vi "RIB Req - UDP Connect.vi"(0 "Limits File Path":path, 5 "Results File Path":path, 11 "error in":errorcluster) -> (4 "Results Data Array":string[][](array[string]), 15 "error out":errorcluster)   [LabVIEW 2024]
doc: "Template test"
uses:
  <vilib>/addons/_JKI Toolkits/State Machine/_JKI_lib_State_Machine.llb/Select State(s)_err__jki_lib_state_machine.vi
  <vilib>/DAQmx/write.llb/DAQmx Write (Digital 1D Bool 1Chan 1Samp).vi
  <vilib>/addons/_JKI Toolkits/State Machine/_JKI_lib_State_Machine.llb/Select State(s)_bool__jki_lib_state_machine.vi
  <vilib>/addons/_JKI Toolkits/State Machine/_JKI_lib_State_Machine.llb/Periodic Trigger__ogtk__JKI-SM__jki_lib_state_machine.vi
  <userlib>/_OpenG.lib/file/file.llb/Strip Path Extension - String__ogtk.vi
  <vilib>/Utility/file.llb/Read Delimited Spreadsheet (string).vi
  <vilib>/Utility/file.llb/Write Delimited Spreadsheet (string).vi
  <vilib>/DAQmx/create/channels.llb/DAQmx Create Channel (DO-Digital Output).vi
  <vilib>/DAQmx/miscellaneous.llb/DAQmx Fill In Error Info.vi
  <userlib>/_OpenG.lib/file/file.llb/openg_file.lvlib
  <userlib>/_OpenG.lib/appcontrol/appcontrol.llb/openg_application_control.lvlib
  <userlib>/_OpenG.lib/time/time.llb/openg_time.lvlib
panel:
  out "Connect":bool
  out "Connect Fail":bool
  out "Timeout (Connect Fail)":dbl(slide) scale=0.0..10.0
  out "Timeout (Connect)":dbl(slide) scale=0.0..10.0
  in  "Connect":string
  in  "Connect Fail":string
  out "Results Data 5":string[](array[string])
  out "Results Data 4":string[](array[string])
  in  "task out":refnum<k21>
  in  "UDP Read":string
  in  "connection ID":refnum<k16>
  in  "Exit":bool
  # "UDP Initialise Test"
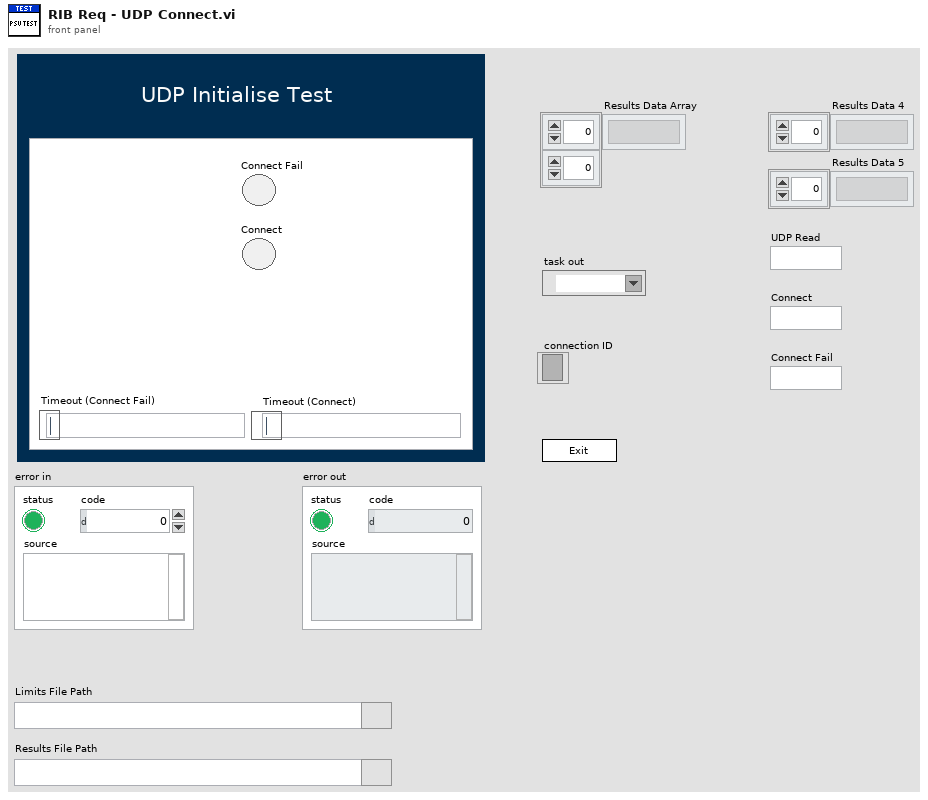
[diagram p1: front panel]
types:
  T1 = enum32{"Invalid", "Standard", "Closed", "Hidden", "Minimized", "Maximized"}
  T2 = enum32{"invalid app kind", "Development System", "Run Time System", "Student Edition", "Embedded LabVIEW", "Evaluation", "Custom"}
  T3 = typedef "FGV - Enum" = enum16{"Cleanup", "Get Data", "Open UDP", "Initialise DAQ", "Initialise I2C"}
  T4 = enum16{"Start Timer", "Get Time", "Pause", "Unpause"}
  T5 = cluster{"Core":cluster{"Current VI Reference":refnum<vi>, "Close Panel on Exit?":bool}, "Limits File Path":path, "Test Limits":string[][], "Results Data Array":string[][], "Results File Path":path, "UDP Read":string, "connection ID":refnum<k16>, "task out":refnum<k21>, "Connect Fail":string, "Connect":string}
  T6 = cluster{"Current VI Reference":refnum<vi>, "Close Panel on Exit?":bool}
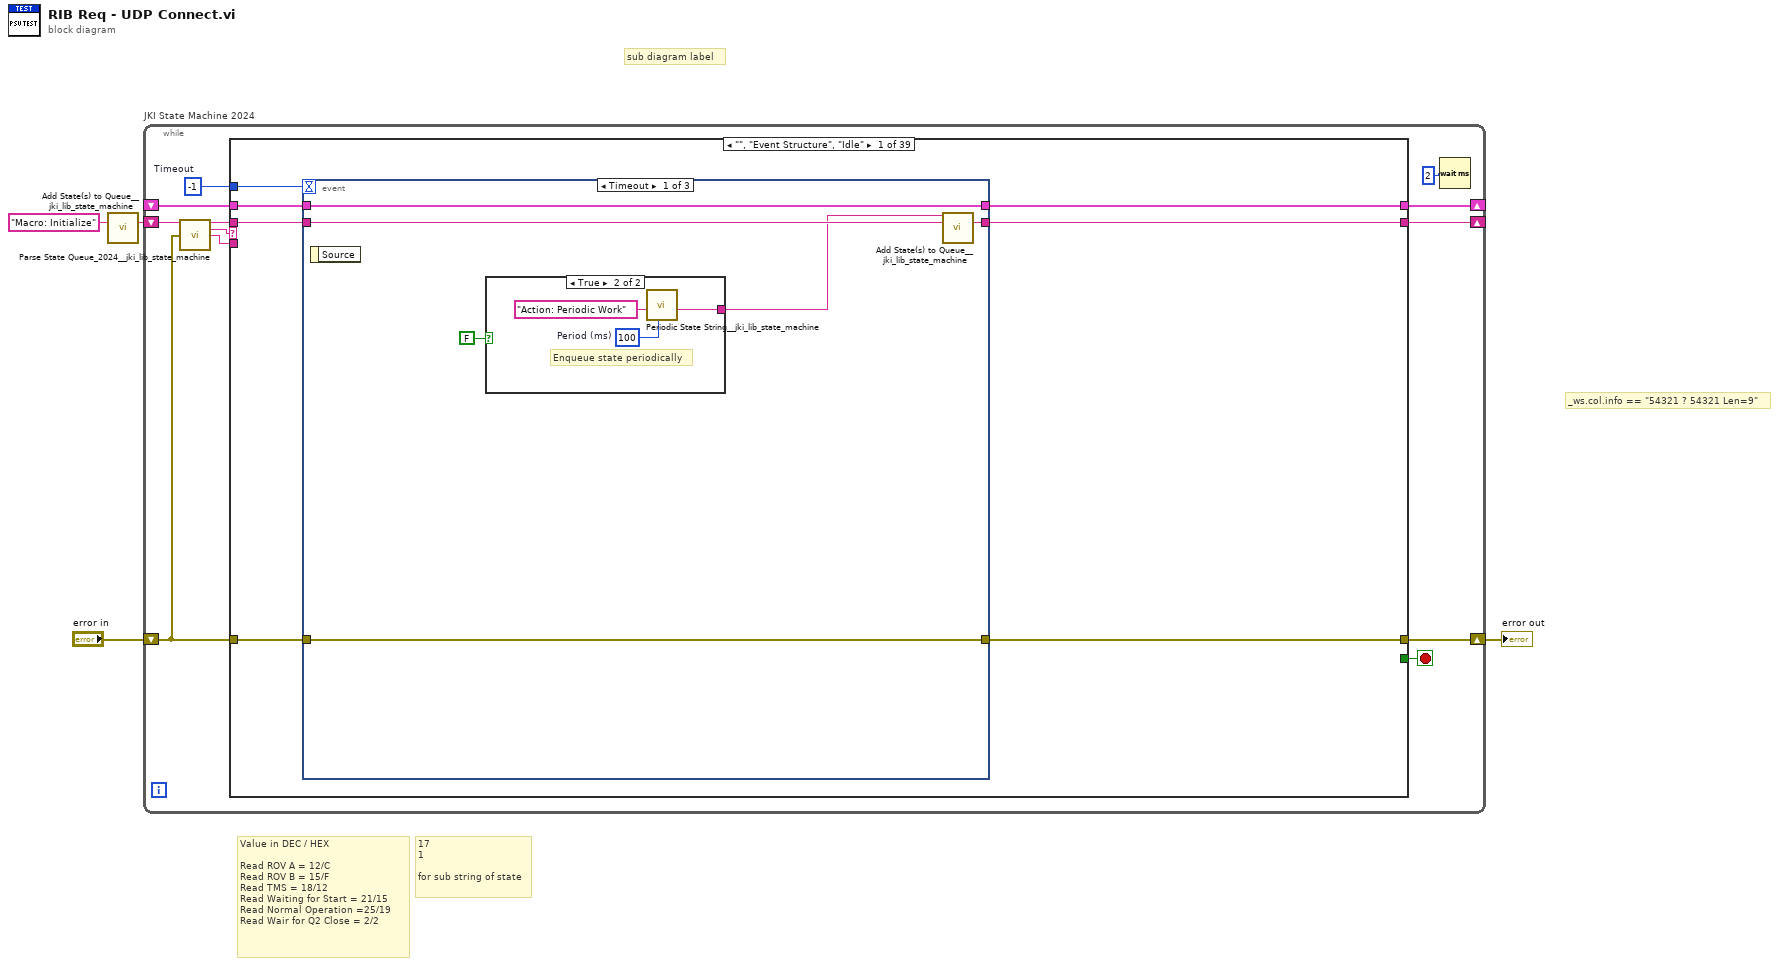
[diagram p0: block diagram]
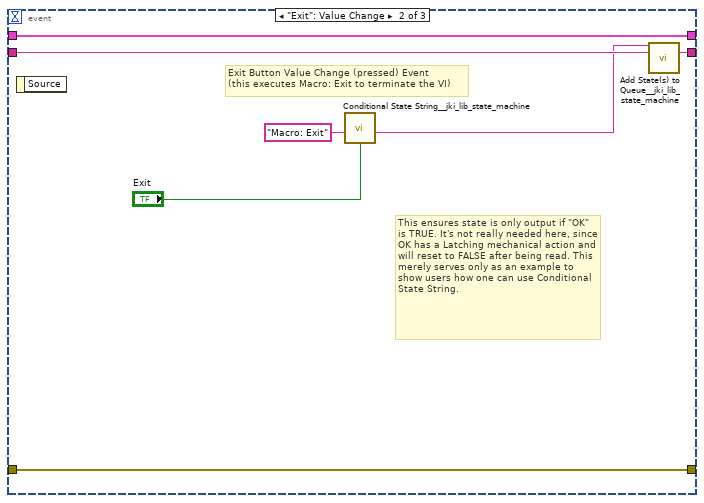
[diagram p3: hidden frame]
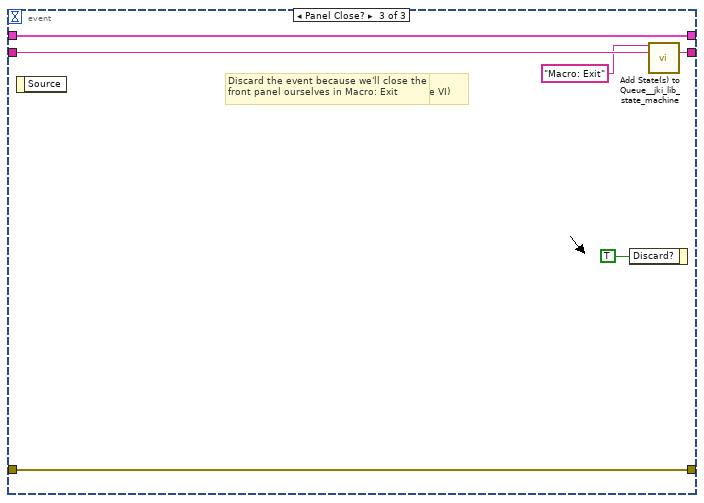
[diagram p4: hidden frame]
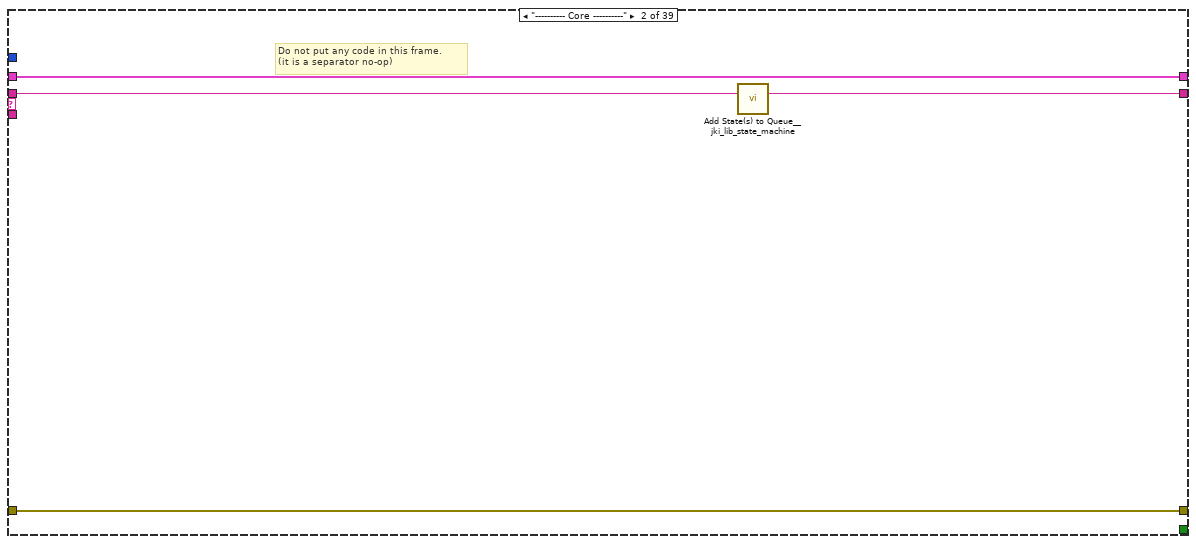
[diagram p5: hidden frame]
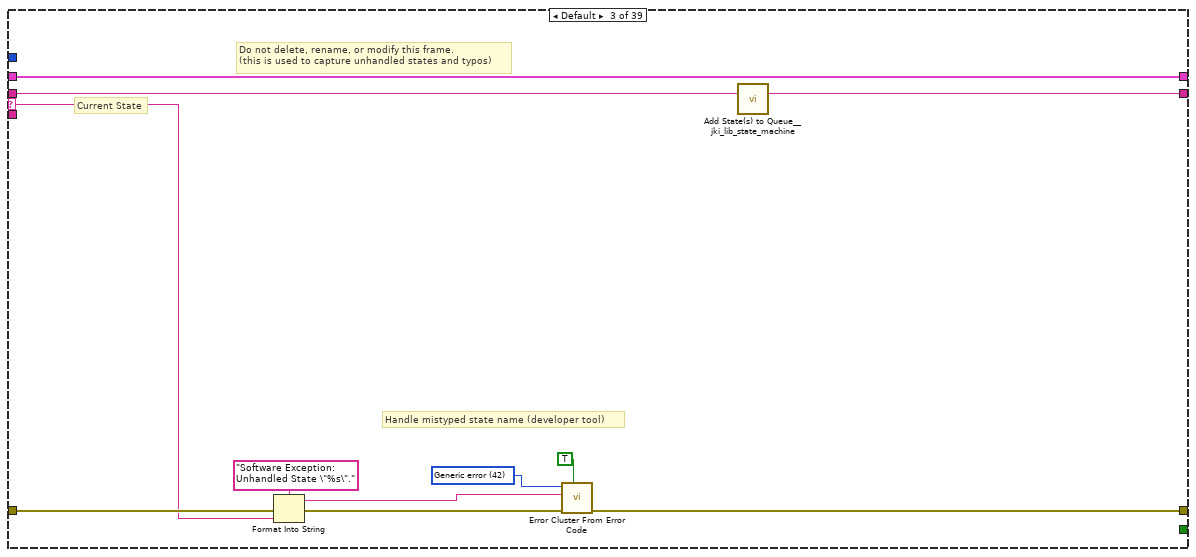
[diagram p6: hidden frame]
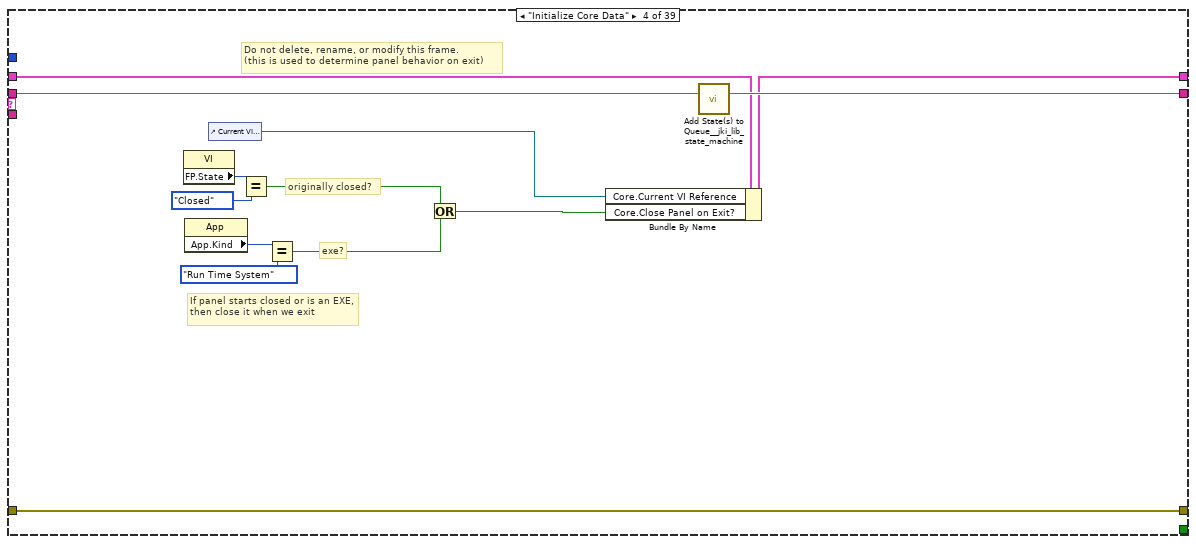
[diagram p7: hidden frame]
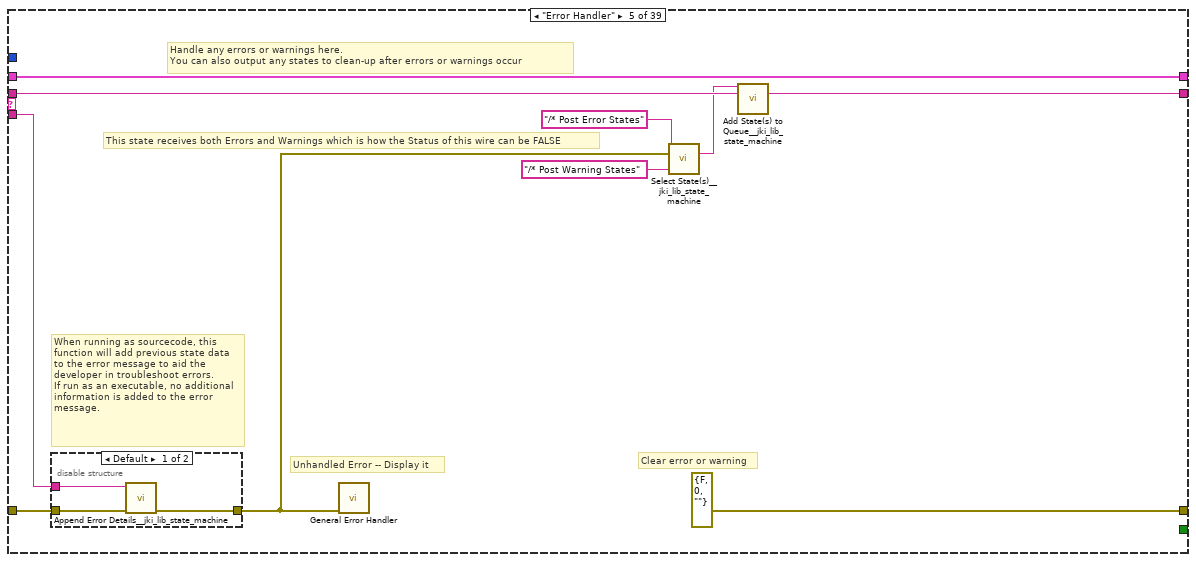
[diagram p8: hidden frame]
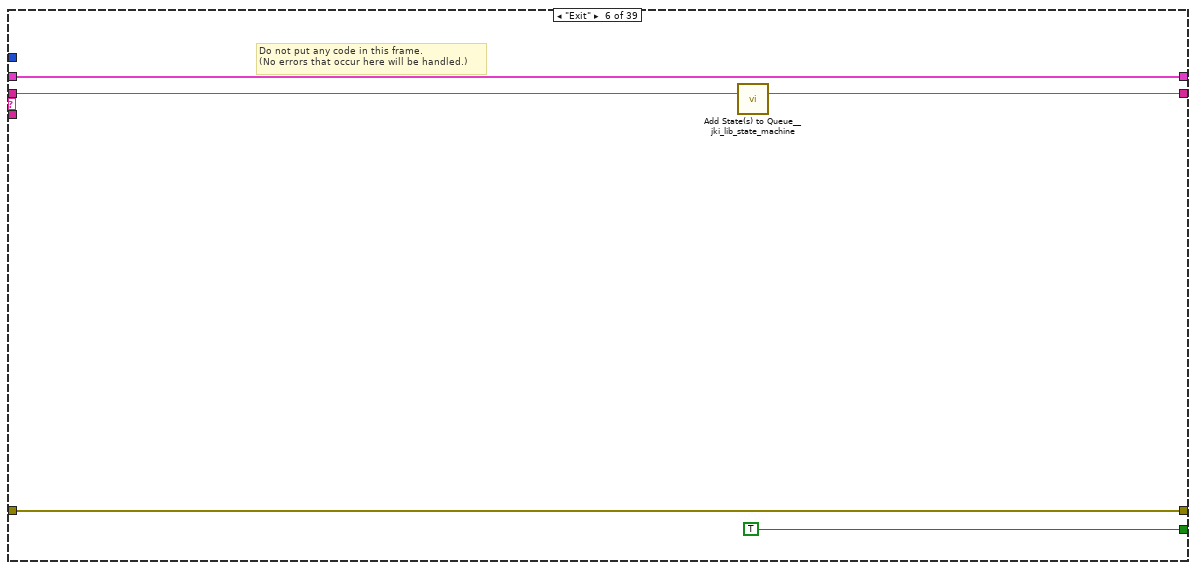
[diagram p10: hidden frame]
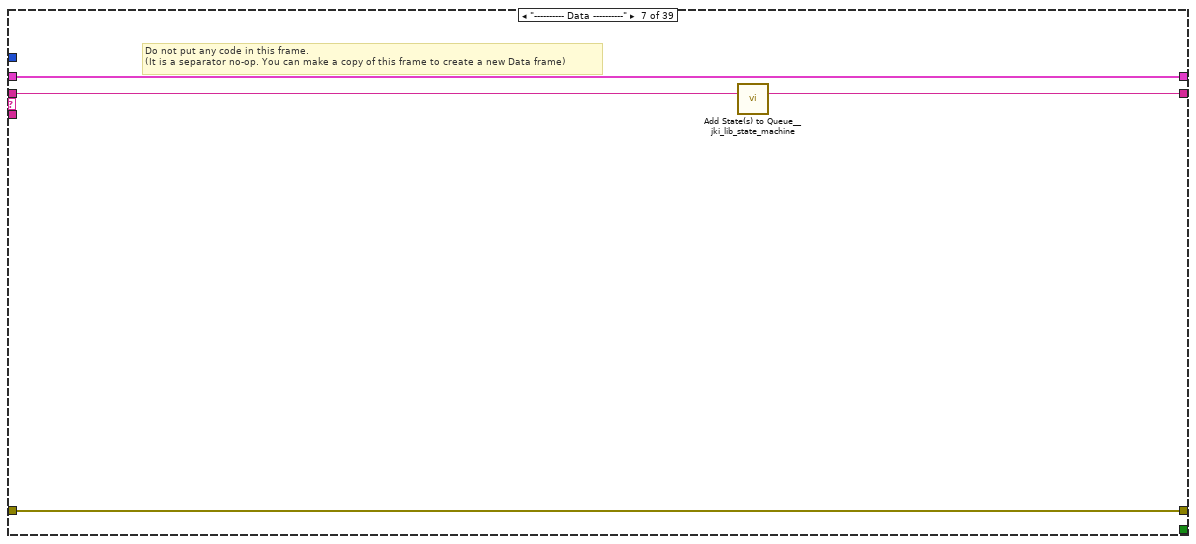
[diagram p11: hidden frame]
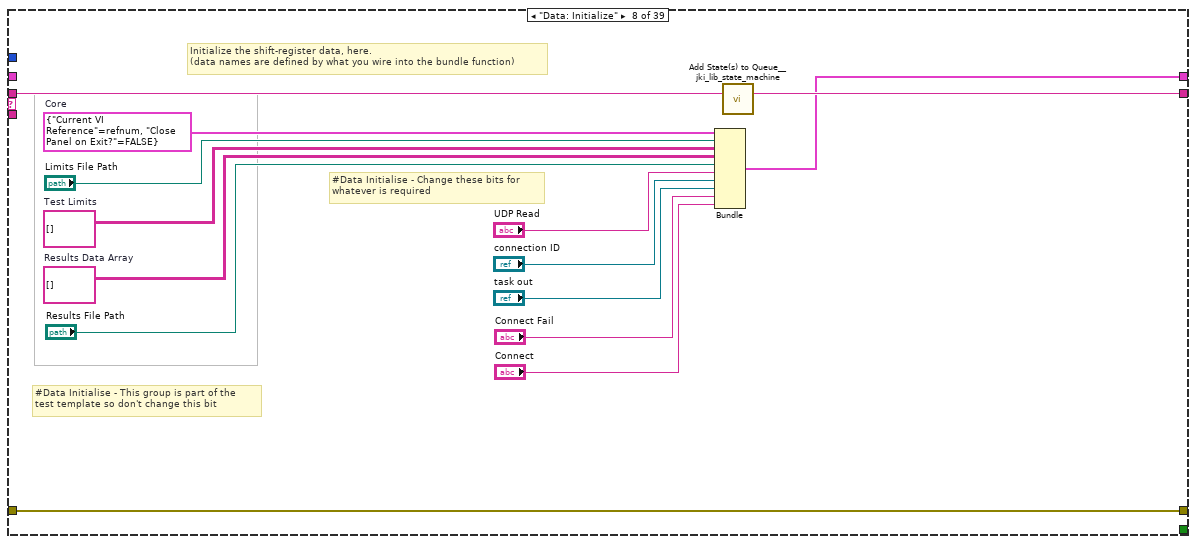
[diagram p12: hidden frame]
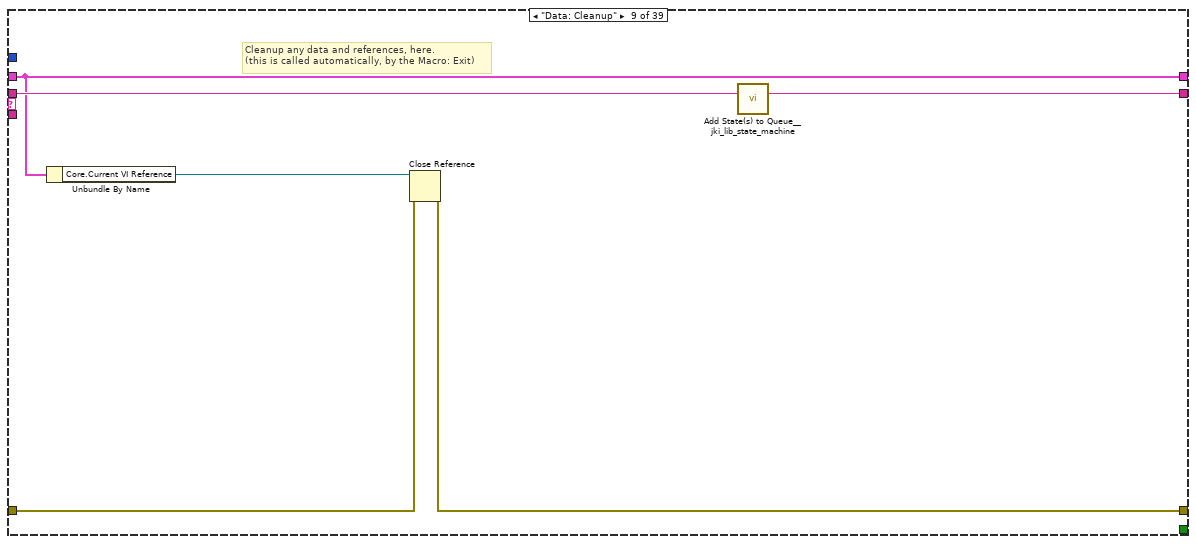
[diagram p13: hidden frame]
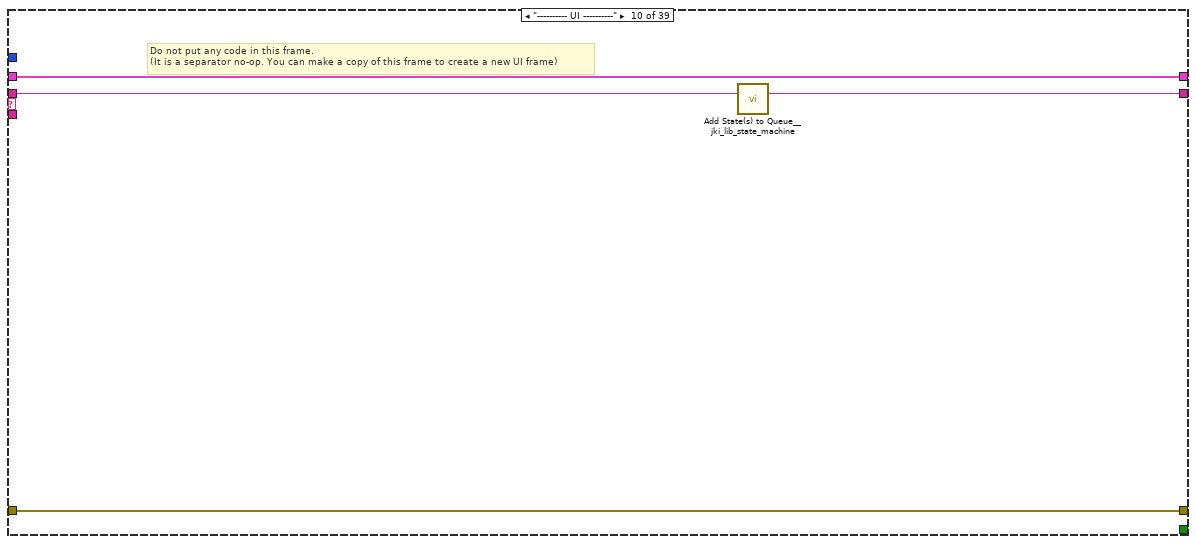
[diagram p14: hidden frame]
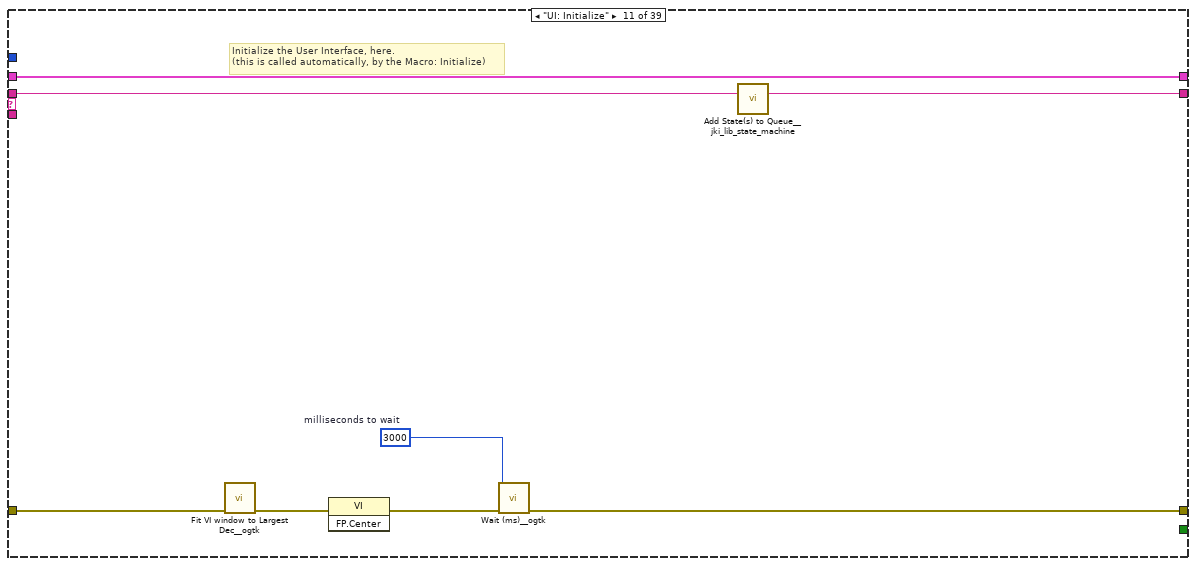
[diagram p15: hidden frame]
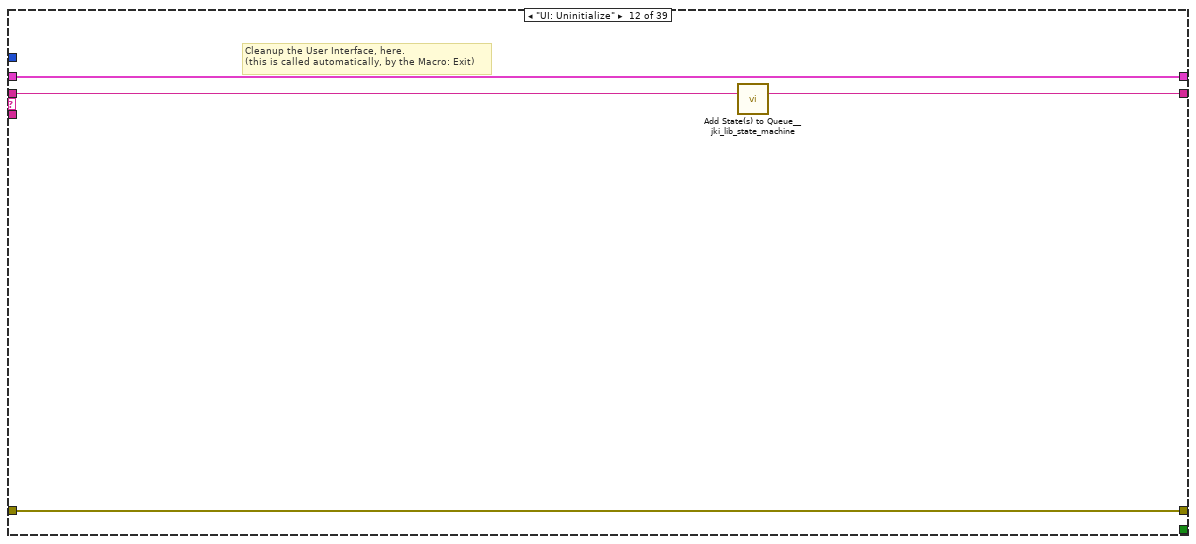
[diagram p16: hidden frame]
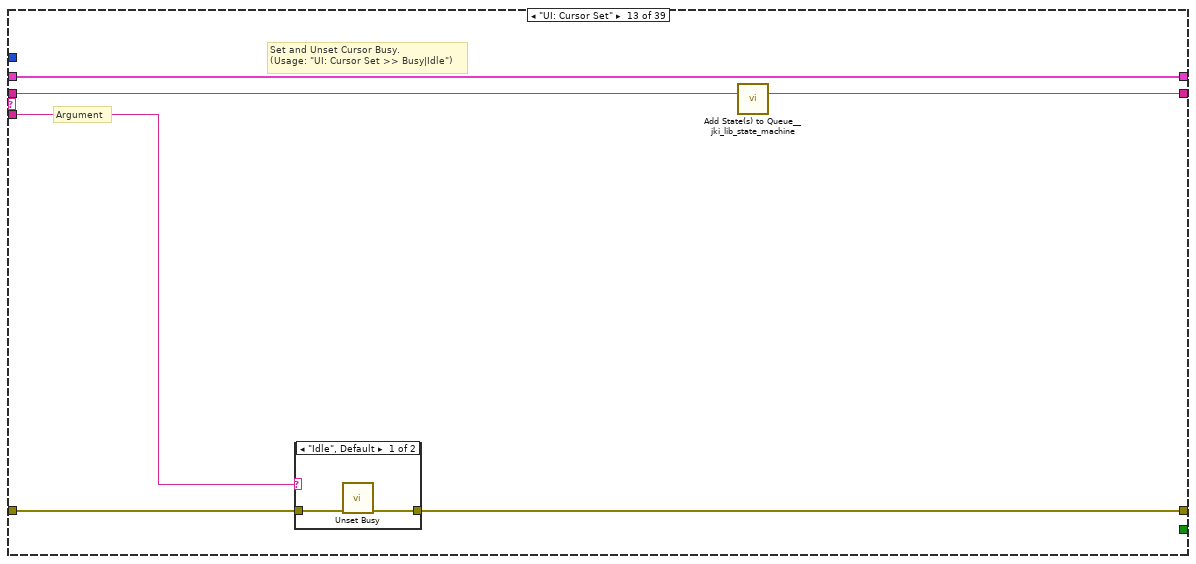
[diagram p17: hidden frame]
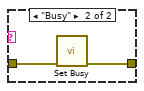
[diagram p18: hidden frame]
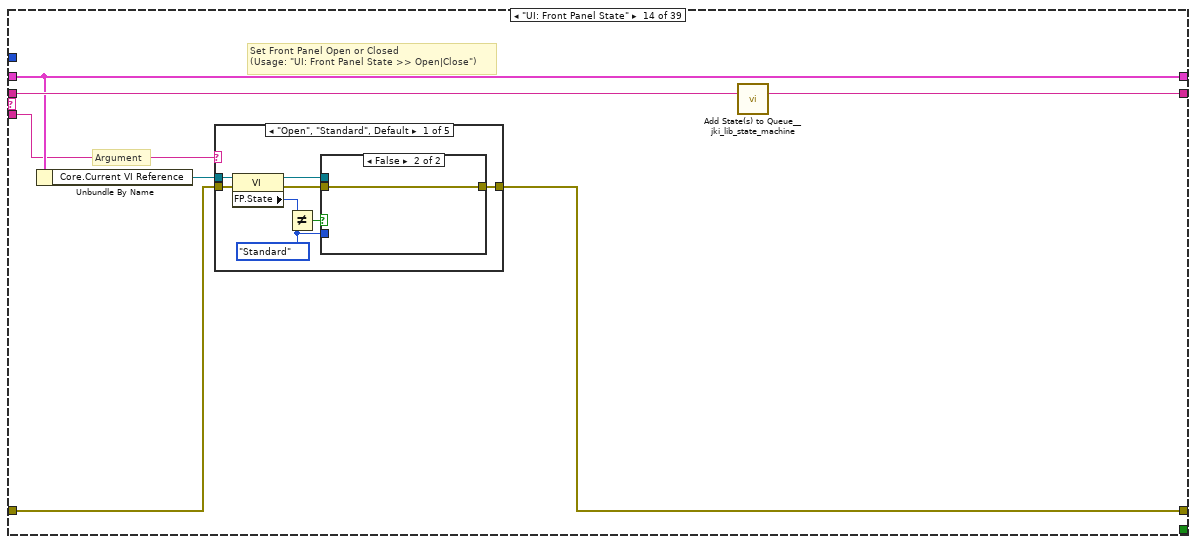
[diagram p19: hidden frame]
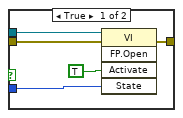
[diagram p20: hidden frame]
diagram:
  # "17\n1\n\nfor sub string of state"
  # "Value in DEC / HEX\n\nRead ROV A = 12/C\nRead ROV B = 15/F\nRead TMS = 18/12\nRead Waiting for Start = 21/15\nRead Normal Operation =25/19 \nRead Wair for Q2 Close = 2/2"
  # "_ws.col.info == \"54321 ? 54321 Len=9\""
  # "sub diagram label"
  n1 = call <vilib>:"Add State(s) to Queue__jki_lib_state_machine.vi"("State(s) in (\"\")"="Macro: Initialize") -> ("States Out"=w4:string)  [unwired: 14 in]
  n2 = while "JKI State Machine 2024" {
    shift-right: [w9] -> _
    shift-left: _ -> [w8]
    shift-right: [w12] -> w1
    shift-left: "error in" -> [w6]
    shift-right: [w11] -> _
    shift-left: w4 -> [w13]
    stop <- w10 stop-if-true
    w7 = -1  # Timeout
    n3 = call <vilib>:"Parse State Queue_2024__jki_lib_state_machine.vi"("State Queue"=w13, "Error In (no error)"=w6) -> ("Remaining States"=w15:string, "Current State"=w16:string, "Arguments"=w14:string)  [unwired: 11 in]
    n4 = case shown="\"\", \"Event Structure\", \"Idle\"" w16 {
      selector: w16 -> [_ _ w50 _ _ _ _ _ _ _ _ _ _ _ _ _ _ _ _ _ _ _ _ _ _ _ _ _ _ _ _ _ _ _ _ _ _ _ _]
      tunnel: w15 -> [w23 w49 w54 w73 w83 w92 w96 w110 w116 w120 w128 w132 w138 w149 w218 w223 w228 w233 w238 w247 w251 w264 w281 w294 w298 w307 w311 w326 w332 w344 w352 w376 w386 w416 w428 w452 w462 w492 w504]
      tunnel: w14 -> [_ _ _ _ w78 _ _ _ _ _ _ _ w133 w143 _ _ _ _ _ _ _ _ _ _ _ _ _ _ _ _ _ _ _ _ _ _ _ _ _]
      tunnel: w8 -> [w21 w46 w52 w66 w80 w90 w93 _ w111 w117 w126 w130 w136 w145 w215 w220 w225 w230 w235 w245 w248 w254 w273 w286 w295 w303 w308 w324 w328 w339 w350 w357 w384 w412 w426 w433 w460 w488 w502]
      tunnel: [w20 w47 w56 w70 errorcluster {"status"=FALSE, "code"=0, "source"=""} ("error out") w89 w94 w107 w112 w118 w124 w129 w134 w146 w216 w221 w226 w231 w236 w242 w249 w260 w278 w291 w296 w305 w309 w314 w327 w335 w347 w354 w377 w407 w423 w430 w453 w484 w499] -> w12
      tunnel: w6 -> [w17 w47 w55 w70 w79 w89 w94 w107 w113 w118 w125 w129 w135 w147 w216 w221 w226 w231 w236 w242 w249 w259 w277 w290 w296 w304 w309 w319 w327 w340 w346 w358 w382 w414 w424 w434 w458 w490 w500]
      tunnel: [w22 w48 w53 w72 w82 w91 w95 w109 w115 w119 w127 w131 w137 w148 w217 w222 w227 w232 w237 w246 w250 w263 w280 w293 w297 w306 w310 w325 w331 w343 w351 w375 w385 w415 w427 w451 w461 w491 w503] -> w11
      tunnel: [_ _ _ _ _ TRUE _ _ _ _ _ _ _ _ _ _ _ _ _ _ _ _ _ _ _ _ _ _ _ _ _ _ _ _ _ _ _ _ _] -> w10
      tunnel: [w19 w46 w52 w71 w80 w90 w93 w108 w111 w117 w126 w130 w136 w145 w215 w220 w225 w230 w235 w245 w248 w253 w272 w285 w295 w303 w308 w324 w328 w338 w349 w359 w384 w411 w426 w435 w460 w487 w502] -> w9
      tunnel: w7 -> [w18 _ _ _ _ _ _ _ _ _ _ _ _ _ _ _ _ _ _ _ _ _ _ _ _ _ _ _ _ _ _ _ _ _ _ _ _ _ _]
      frame "", "Event Structure", "Idle" {
        n5 = event shown="[0] Timeout" {
          selector: _ -> [_ _ _]
          dyn-events: _ -> [_ _ _]
          timeout: w18 -> [_ _ _]
          tunnel: w23 -> [w29 w39 w45]
          tunnel: [w28 w38 w44] -> w22
          tunnel: w21 -> [w26 w36 w42]
          tunnel: [w27 w37 w43] -> w20
          tunnel: w17 -> [w27 w37 w43]
          tunnel: [w26 w36 w42] -> w19
          event Timeout {
            n6 = event-data() -> ()  [unwired: 1 in, 1 out]
            n7 = case shown="True" FALSE {
              tunnel: [_ w32] -> w25
              frame False {
              }
              frame True {
                w30 = u32 100  # Period (ms)
                # "Enqueue state periodically"
                n8 = call <vilib>:"Periodic State String__jki_lib_state_machine.vi"("Period (ms)"=w30, "State"="Action: Periodic Work") -> ("State Out"=w32:string)  [unwired: 9 in]
              }
            }
            n9 = call <vilib>:"Add State(s) to Queue__jki_lib_state_machine.vi"("State(s) in Front (\"\")"=w25, "State(s) in (\"\")"=w29) -> ("States Out"=w28:string)  [unwired: 13 in]
          }
          event "Exit": Value Change {
            # "This ensures state is only output if \"OK\" is TRUE. It's not really needed here, since OK has a Latching mechanical action and will reset to FALSE after being read. This merely serves only as an example to show users how one can use Conditional State String."
            # "Exit Button Value Change (pressed) Event\n(this executes Macro: Exit to terminate the VI)"
            n10 = event-data() -> ()  [unwired: 1 in, 1 out]
            n11 = call <vilib>:"Conditional State String__jki_lib_state_machine.vi"("Do State(s)?"="Exit", "State"="Macro: Exit") -> ("State Out"=w33:string)  [unwired: 7 in]
            n12 = call <vilib>:"Add State(s) to Queue__jki_lib_state_machine.vi"("State(s) in Front (\"\")"=w33, "State(s) in (\"\")"=w39) -> ("States Out"=w38:string)  [unwired: 13 in]
          }
          event Panel Close? {
            # "Discard the event because we'll close the front panel ourselves in Macro: Exit"
            # "Close Panel button (pressed) Event\n(this executes Macro: Exit to terminate the VI)"
            n13 = event-data() -> ()  [unwired: 1 in, 1 out]
            n14 = event-data("Discard?"=TRUE) -> ()  [unwired: 1 in, 1 out]
            n15 = call <vilib>:"Add State(s) to Queue__jki_lib_state_machine.vi"("State(s) in Front (\"\")"="Macro: Exit", "State(s) in (\"\")"=w45) -> ("States Out"=w44:string)  [unwired: 13 in]
          }
        }
      }
      frame "---------- Core ----------" {
        # "Do not put any code in this frame.\n(it is a separator no-op)"
        n16 = call <vilib>:"Add State(s) to Queue__jki_lib_state_machine.vi"("State(s) in (\"\")"=w49) -> ("States Out"=w48:string)  [unwired: 14 in]
      }
      frame Default {
        w59 = 42 items=["No error", "Argument error", "Memory is full", "Out of zone", "End of file", "File already open", "Generic file I/O error", "File not found", "File permission error", "Disk is full", "Duplicate path", "Too many files open", "System feature not enabled", "Resource file not found", "Cannot add resource", "Resource not found", "Image not found", "Image memory error", "Pen does not exist", "Config type invalid", "Config token not found", "Config parse error", "Config memory error", "Bad external code format", "Bad external code offset", "External code not present", "Null window", "Destroy window error", "Null menu", "Print aborted", "Bad print record", "Print driver error", "Windows error during printing", "Memory error during printing", "Print dialog error", "Generic print error", "Invalid device refnum", "Device not found", "Device parameter error", "Device unit error", "Cannot open device", "Device call aborted", "Generic error", "Cancelled by user", "Object ID too low", "Object ID too high", "Object not in heap", "Unknown heap", "Unknown object (invalid DefProc)", "Unknown object (DefProc not in table)", "Message out of range", "Invalid (null) method", "Unknown message", "Manager call not supported", "Bad address", "Network operation in progress", "Network operation timed out", "Connection is busy", "Network attribute not supported", "Network error", "Address in use", "System out of memory", "Connection aborted", "Connection refused", "Not connected", "Already connected", "Connection closed", "Initialization error (interapplication manager)", "Bad occurrence", "Wait on unbound occurrence handler", "Occurrence queue overflow", "Datalog type conflict", "Unused", "Unrecognized type (interapplication manager)", "Memory corrupt", "Failed to make temporary DLL", "Old CIN version", "Drag socket not found", "Failed to load drop-object", "Failed to register OLE object", "Failed to release OLE object", "Format specifier type mismatch", "Unknown format specifier", "Too few format specifiers", "Too many format specifiers", "Scan failed", "Newer CIN version", "Error converting to variant", "Runtime menu error", "Password tampered", "Variant attribute not found", "Incompatible variant data type", "Event data is not available", "Event Store is not present", "Occurrence is not found", "Event Queue is not created", "Event info is not available", "Refnum passed is NULL", "Error retrieving Class GUID", "Error retrieving CoClass GUID", "Error retrieving TypeLib GUID.", "Bad built application magic bytes.", "Specific driver is different from the specific driver associated with the Logical Name.", "There is no session opened to the class driver.", "Max Error", "MAX - Error with config objects", "MAX - Error loading configuration", "MAX - Group not supported"]
        # "Current State"
        # "Do not delete, rename, or modify this frame.\n(this is used to capture unhandled states and typos)"
        # "Handle mistyped state name (developer tool)"
        n17 = Format Into String(format string="Software Exception: Unhandled State \"%s\"." ("message"), error in=w55, w50) -> (resulting string=w58:string, error out=w57:errorcluster)  [unwired: 1 in]
        n18 = call <vilib>:"Error Cluster From Error Code.vi"("show call chain? (False)"=TRUE, "error in (no error)"=w57, "error message (\"\")"=w58, "error code (0)"=w59) -> ("error out"=w56:errorcluster)  [unwired: 5 in]
        n19 = call <vilib>:"Add State(s) to Queue__jki_lib_state_machine.vi"("State(s) in (\"\")"=w54) -> ("States Out"=w53:string)  [unwired: 14 in]
      }
      frame "Initialize Core Data" {
        # "Do not delete, rename, or modify this frame.\n(this is used to determine panel behavior on exit)"
        # "originally closed?"
        # "exe?"
        # "If panel starts closed or is an EXE, then close it when we exit"
        n20 = property class="VI"() -> ("FP.State"=w63:T1)  [unwired: 2 in, 2 out]
        n21 = property class="App"() -> ("App.Kind"=w69:T2)  [unwired: 2 in, 2 out]
        n22 = control-ref of="Current VI Reference"() -> (w64:refnum<vi>)
        n23 = Equal?(x=w63, y=T1."Closed" ("Front Panel Window:State")) -> (x = y?=w61:bool)
        n24 = Equal?(x=w69, y=T2."Run Time System" ("Application:Kind")) -> (x = y?=w67:bool)
        n25 = Or(x=w61, y=w67) -> (x .or. y?=w65:bool)
        n26 = Bundle By Name(cluster=w66, "Core.Current VI Reference"=w64, "Core.Close Panel on Exit?"=w65) -> (w71:T5)
        n27 = call <vilib>:"Add State(s) to Queue__jki_lib_state_machine.vi"("State(s) in (\"\")"=w73) -> ("States Out"=w72:string)  [unwired: 14 in]
      }
      frame "Error Handler" {
        # "When running as sourcecode, this function will add previous state data to the error message to aid the developer in troubleshoot errors.\nIf run as an executable, no additional information is added to the error message."
        # "This state receives both Errors and Warnings which is how the Status of this wire can be FALSE"
        # "Unhandled Error -- Display it"
        # "Handle any errors or warnings here.\nYou can also output any states to clean-up after errors or warnings occur"
        # "Clear error or warning"
        n28 = disable-structure shown="Default" {
          disable-tunnel: w79 -> [w86 w87]
          disable-tunnel: w78 -> [w85 _]
          disable-tunnel: [w84 w87] -> w77
          frame condition #0 (active) {
            n29 = call <vilib>:"Append Error Details__jki_lib_state_machine.vi"("error in (no error)"=w86, "Previous State and Argument(s)"=w85) -> ("error out"=w84:errorcluster)  [unwired: 9 in]
          }
          frame condition #1 {
          }
        }
        n30 = call <vilib>:"General Error Handler.vi"("error in (no error)"=w77) -> ()  [unwired: 10 in, 5 out]
        n31 = call-poly <vilib>:"Select State(s)__jki_lib_state_machine.vi"("State(s) if True (\"\")"="/* Post Error States", "Select"=w77, "State(s) if False (\"\")"="/* Post Warning States") -> ("States Out"=w75:string)  [unwired: 12 in]
        n32 = call <vilib>:"Add State(s) to Queue__jki_lib_state_machine.vi"("State(s) in Front (\"\")"=w75, "State(s) in (\"\")"=w83) -> ("States Out"=w82:string)  [unwired: 13 in]
      }
      frame "Exit" {
        # "Do not put any code in this frame.\n(No errors that occur here will be handled.)"
        n33 = call <vilib>:"Add State(s) to Queue__jki_lib_state_machine.vi"("State(s) in (\"\")"=w92) -> ("States Out"=w91:string)  [unwired: 14 in]
      }
      frame "---------- Data ----------" {
        # "Do not put any code in this frame.\n(It is a separator no-op. You can make a copy of this frame to create a new Data frame)"
        n34 = call <vilib>:"Add State(s) to Queue__jki_lib_state_machine.vi"("State(s) in (\"\")"=w96) -> ("States Out"=w95:string)  [unwired: 14 in]
      }
      frame "Data: Initialize" {
        w103 = string[][] []  # Results Data Array
        w104 = string[][] []  # Test Limits
        w106 = T6 {"Current VI Reference"=refnum, "Close Panel on Exit?"=FALSE}  # Core
        # "#Data Initialise - Change these bits for\nwhatever is required"
        # "#Data Initialise - This group is part of the\ntest template so don't change this bit"
        # "Initialize the shift-register data, here.\n(data names are defined by what you wire into the bundle function)"
        n35 = Bundle("Core"=w106, "Limits File Path"="Limits File Path", "Test Limits"=w104, "Results Data Array"=w103, "Results File Path"="Results File Path", "UDP Read"="UDP Read", "connection ID"="connection ID", "task out"="task out", "Connect Fail"="Connect Fail", "Connect"="Connect") -> (w108:T5)  [unwired: 1 in]
        n36 = call <vilib>:"Add State(s) to Queue__jki_lib_state_machine.vi"("State(s) in (\"\")"=w110) -> ("States Out"=w109:string)  [unwired: 14 in]
      }
      frame "Data: Cleanup" {
        # "Cleanup any data and references, here.\n(this is called automatically, by the Macro: Exit)"
        n37 = Unbundle By Name(w111) -> ("Core.Current VI Reference"=w114:refnum<vi>)
        n38 = Close Reference(reference=w114, error in (no error)=w113) -> (error out=w112:errorcluster)
        n39 = call <vilib>:"Add State(s) to Queue__jki_lib_state_machine.vi"("State(s) in (\"\")"=w116) -> ("States Out"=w115:string)  [unwired: 14 in]
      }
      frame "---------- UI ----------" {
        # "Do not put any code in this frame.\n(It is a separator no-op. You can make a copy of this frame to create a new UI frame)"
        n40 = call <vilib>:"Add State(s) to Queue__jki_lib_state_machine.vi"("State(s) in (\"\")"=w120) -> ("States Out"=w119:string)  [unwired: 14 in]
      }
      frame "UI: Initialize" {
        w123 = u32 3000  # milliseconds to wait
        # "Initialize the User Interface, here.\n(this is called automatically, by the Macro: Initialize)"
        n41 = call <userlib>:"Fit VI window to Largest Dec__ogtk.vi"("error in (no error)"=w125) -> ("error out"=w121:errorcluster)  [unwired: 5 in, 1 out]
        n42 = invoke class="VI" method="FP.Center"(error in=w121) -> (error out=w122:errorcluster)  [unwired: 2 in, 2 out]
        n43 = call <userlib>:"Wait (ms)__ogtk.vi"("error in (no error)"=w122, "milliseconds to wait"=w123) -> ("error out"=w124:errorcluster)  [unwired: 8 in, 1 out]
        n44 = call <vilib>:"Add State(s) to Queue__jki_lib_state_machine.vi"("State(s) in (\"\")"=w128) -> ("States Out"=w127:string)  [unwired: 14 in]
      }
      frame "UI: Uninitialize" {
        # "Cleanup the User Interface, here.\n(this is called automatically, by the Macro: Exit)"
        n45 = call <vilib>:"Add State(s) to Queue__jki_lib_state_machine.vi"("State(s) in (\"\")"=w132) -> ("States Out"=w131:string)  [unwired: 14 in]
      }
      frame "UI: Cursor Set" {
        # "Argument"
        # "Set and Unset Cursor Busy.\n(Usage: \"UI: Cursor Set >> Busy|Idle\")"
        n46 = case shown="\"Idle\", Default" w133 {
          tunnel: w135 -> [w140 w142]
          tunnel: [w139 w141] -> w134
          frame "Idle", Default {
            n47 = call <vilib>:"Unset Busy.vi"("error in (no error)"=w140) -> ("error out"=w139:errorcluster)  [unwired: 10 in]
          }
          frame "Busy" {
            n48 = call <vilib>:"Set Busy.vi"("error in (no error)"=w142) -> ("error out"=w141:errorcluster)  [unwired: 9 in, 1 out]
          }
        }
        n49 = call <vilib>:"Add State(s) to Queue__jki_lib_state_machine.vi"("State(s) in (\"\")"=w138) -> ("States Out"=w137:string)  [unwired: 14 in]
      }
      frame "UI: Front Panel State" {
        # "Argument"
        # "Set Front Panel Open or Closed\n(Usage: \"UI: Front Panel State >> Open|Close\")"
        n50 = Unbundle By Name(w145) -> ("Core.Current VI Reference"=w144:refnum<vi>)
        n51 = case shown="\"Open\", \"Standard\", Default" w143 {
          tunnel: w147 -> [w155 w170 w181 w194 w207]
          tunnel: [w157 w171 w183 w196 w209] -> w146
          tunnel: w144 -> [w156 w168 w182 w195 w208]
          frame "Open", "Standard", Default {
            w150 = T1."Standard" ("State")
            n52 = property class="VI"(reference=w156, error in=w155) -> (reference out=w153:refnum<vi>, error out=w154:errorcluster, "FP.State"=w152:T1)
            n53 = Not Equal?(x=w152, y=w150) -> (x != y?=w151:bool)
            n54 = case shown="False" w151 {
              tunnel: [w161 w163] -> w157
              tunnel: w154 -> [w160 w163]
              tunnel: w153 -> [w159 _]
              tunnel: w150 -> [w158 _]
              frame True {
                n55 = invoke class="VI" method="FP.Open"(reference=w159, error in=w160, "Activate"=TRUE, "State"=w158) -> (error out=w161:errorcluster)  [unwired: 1 in, 4 out]
              }
              frame False {
              }
            }
          }
          frame "Close", "Closed" {
            n56 = property class="VI"(reference=w168, error in=w170) -> (reference out=w167:refnum<vi>, error out=w169:errorcluster, "FP.State"=w165:T1)
            n57 = Not Equal?(x=w165, y=T1."Closed" ("Front Panel Window:State")) -> (x != y?=w164:bool)
            n58 = case shown="True" w164 {
              tunnel: [w172 w175] -> w171
              tunnel: w169 -> [w172 w174]
              tunnel: w167 -> [_ w173]
              frame False {
              }
              frame True {
                n59 = invoke class="VI" method="FP.Close"(reference=w173, error in=w174) -> (error out=w175:errorcluster)  [unwired: 1 in, 2 out]
              }
            }
          }
          frame "Hidden", "Hide" {
            w176 = T1."Hidden" ("State")
            n60 = property class="VI"(reference=w182, error in=w181) -> (reference out=w179:refnum<vi>, error out=w180:errorcluster, "FP.State"=w178:T1)
            n61 = Not Equal?(x=w178, y=w176) -> (x != y?=w177:bool)
            n62 = case shown="True" w177 {
              tunnel: [w187 w188] -> w183
              tunnel: w180 -> [w186 w188]
              tunnel: w179 -> [w185 _]
              tunnel: w176 -> [w184 _]
              frame True {
                n63 = invoke class="VI" method="FP.Open"(reference=w185, error in=w186, "State"=w184) -> (error out=w187:errorcluster)  [unwired: 2 in, 4 out]
              }
              frame False {
              }
            }
          }
          frame "Minimize", "Minimized" {
            w189 = T1."Minimized" ("State")
            n64 = property class="VI"(reference=w195, error in=w194) -> (reference out=w192:refnum<vi>, error out=w193:errorcluster, "FP.State"=w191:T1)
            n65 = Not Equal?(x=w191, y=w189) -> (x != y?=w190:bool)
            n66 = case shown="True" w190 {
              tunnel: [w200 w201] -> w196
              tunnel: w193 -> [w199 w201]
              tunnel: w192 -> [w198 _]
              tunnel: w189 -> [w197 _]
              frame True {
                n67 = invoke class="VI" method="FP.Open"(reference=w198, error in=w199, "State"=w197) -> (error out=w200:errorcluster)  [unwired: 2 in, 4 out]
              }
              frame False {
              }
            }
          }
          frame "Maximize", "Maximized" {
            w202 = T1."Maximized" ("State")
            n68 = property class="VI"(reference=w208, error in=w207) -> (reference out=w205:refnum<vi>, error out=w206:errorcluster, "FP.State"=w204:T1)
            n69 = Not Equal?(x=w204, y=w202) -> (x != y?=w203:bool)
            n70 = case shown="True" w203 {
              tunnel: [w213 w214] -> w209
              tunnel: w206 -> [w212 w214]
              tunnel: w205 -> [w211 _]
              tunnel: w202 -> [w210 _]
              frame True {
                n71 = invoke class="VI" method="FP.Open"(reference=w211, error in=w212, "State"=w210) -> (error out=w213:errorcluster)  [unwired: 2 in, 4 out]
              }
              frame False {
              }
            }
          }
        }
        n72 = call <vilib>:"Add State(s) to Queue__jki_lib_state_machine.vi"("State(s) in (\"\")"=w149) -> ("States Out"=w148:string)  [unwired: 14 in]
      }
      frame "---------- Macro ----------" {
        # "Do not put any code in this frame.\n(It is a separator no-op. You can make a copy of this frame to create a new Macro frame)"
        n73 = call <vilib>:"Add State(s) to Queue__jki_lib_state_machine.vi"("State(s) in (\"\")"=w218) -> ("States Out"=w217:string)  [unwired: 14 in]
      }
      frame "Macro: Initialize" {
        # "Initialization Macro\n(This is called once, when the VI starts)"
        n74 = call <vilib>:"Add State(s) to Queue__jki_lib_state_machine.vi"("State(s) in Front (\"\")"="Data: Initialize\nInitialize Core Data\nUI: Initialize\nUI: Front Panel State >> Open\nMacro: Test", "State(s) in (\"\")"=w223) -> ("States Out"=w222:string)  [unwired: 13 in]
      }
      frame "Macro: Test" {
        # "#Test Macro - Add the sequence \nfor measurments and limits testing here"
        n75 = call <vilib>:"Add State(s) to Queue__jki_lib_state_machine.vi"("State(s) in Front (\"\")"="Limits Test: Read Limits File\nConnect: Switch Contactor\nConnect: Set IP Address\nConnect: UDP Open\nConnect: UPD Connect Fail\nConnect: Start Timer (Connect Fail)\nConnect: Read Connect Fail", "State(s) in (\"\")"=w228) -> ("States Out"=w227:string)  [unwired: 13 in]
      }
      frame "Macro: Test 2" {
        # "#Test Macro - Add the sequence \nfor measurments and limits testing here"
        n76 = call <vilib>:"Add State(s) to Queue__jki_lib_state_machine.vi"("State(s) in Front (\"\")"="Connect: UPD Connect\nConnect: Start Timer (Connect)\nConnect: Read Connect", "State(s) in (\"\")"=w233) -> ("States Out"=w232:string)  [unwired: 13 in]
      }
      frame "Macro: Limits" {
        # "Do not put any code in this frame.\n(It is a separator no-op. You can make a copy of this frame to create a new Macro frame)"
        n77 = call <vilib>:"Add State(s) to Queue__jki_lib_state_machine.vi"("State(s) in Front (\"\")"="Limits Test: Connect Fail Test\nLimits Test: Connect Test\nResults Data: Write Results Data\nMacro: Exit", "State(s) in (\"\")"=w238) -> ("States Out"=w237:string)  [unwired: 13 in]
      }
      frame "Macro: Exit" {
        # "Exit Macro\n(This is called once, when the VI exits)"
        n78 = Unbundle By Name(w245) -> ("Core.Close Panel on Exit?"=w240:bool)
        n79 = call <vilib>:"Conditional State String__jki_lib_state_machine.vi"("Do State(s)?"=w240, "State"="UI: Front Panel State >> Close") -> ("State Out"=w239:string)  [unwired: 7 in]
        n80 = call <vilib>:"Add State(s) to Queue__jki_lib_state_machine.vi"("State(s) in (\"\")"=w239, "State(s) at Back (\"\")"="UI: Uninitialize\nData: Cleanup\nExit") -> ("States Out"=w243:string)  [unwired: 13 in]
        n81 = call <vilib>:"Add State(s) to Queue__jki_lib_state_machine.vi"("State(s) in Front (\"\")"=w243, "State(s) in (\"\")"=w247) -> ("States Out"=w246:string)  [unwired: 13 in]
      }
      frame "---------- Limits Test ----------" {
        # "Template Separator\n(You can make a copy of, or modify, this frame)"
        n82 = call <vilib>:"Add State(s) to Queue__jki_lib_state_machine.vi"("State(s) in (\"\")"=w251) -> ("States Out"=w250:string)  [unwired: 14 in]
      }
      frame "Limits Test: Read Limits File" {
        w257 = ","  # delimiter (\t)
        n83 = Unbundle By Name(w254) -> ("Limits File Path"=w258:path)
        n84 = Current VI's Path "Test Case Path"() -> (path=w262:path)
        n85 = call-poly <vilib>:"Read Delimited Spreadsheet.vi"("file path (dialog if empty)"=w258, "error in (no error)"=w259, "delimiter (\\t)"=w257) -> ("all rows"=w255:string[][], "error out"=w260:errorcluster)  [unwired: 7 in, 4 out]
        n86 = Strip Path(path=w262) -> (name=w261:string)  [unwired: 1 out]
        n87 = call-poly <userlib>:"Strip Path Extension__ogtk.vi"("path"=w261) -> ("root"=w256:string)  [unwired: 1 out]
        n88 = for {
          tunnel: w256 -> [w268]
          tunnel: w255 -> [w266] mode=indexing
          tunnel: [w266] -> w252 mode=indexing if=w265
          n89 = Index Array(array=w266) -> (element=w267:string)  [unwired: 1 in]
          n90 = Equal?(x=w268, y=w267) -> (x = y?=w265:bool)
        }
        n91 = Bundle By Name(cluster=w254, "Test Limits"=w252) -> (w253:T5)
        n92 = call <vilib>:"Add State(s) to Queue__jki_lib_state_machine.vi"("State(s) in (\"\")"=w264) -> ("States Out"=w263:string)  [unwired: 14 in]
      }
      frame "Limits Test: Connect Fail Test" {
        w274 = "Connect Fail Test"  # Sub Test Name
        # "UDP Read Test = if equal to F0 = pass else fail"
        # "#Limits Testing - Add the sub test name for\ntest included in limits file"
        n93 = Unbundle By Name(w273) -> ("Test Limits"=w275:string[][], "Connect Fail"=w279:string)
        n94 = Unbundle By Name(w273) -> ("Results Data Array"=w271:string[][])
        n95 = To Variant(anything=w279) -> (Variant=w276:variant)
        n96 = call "Process Results.vi"("error in (no error)"=w277, "Measurement"=w276, "Test Limits"=w275, "Sub Test Name"=w274) -> ("error out"=w278:errorcluster, "Results Data"=w269:string[])  [unwired: 6 in]
        "Results Data 4" <- w269
        n97 = Build Array (concatenate)(w271, w269) -> (w270:string[][])
        n98 = Bundle By Name(cluster=w273, "Results Data Array"=w270) -> (w272:T5)
        n99 = call <vilib>:"Add State(s) to Queue__jki_lib_state_machine.vi"("State(s) in (\"\")"=w281) -> ("States Out"=w280:string)  [unwired: 14 in]
      }
      frame "Limits Test: Connect Test" {
        w287 = "Connect Test"  # Sub Test Name
        # "UDP Read Test = if equal to F0 = pass else fail"
        # "#Limits Testing - Add the sub test name for\ntest included in limits file"
        n100 = Unbundle By Name(w286) -> ("Results Data Array"=w284:string[][])
        n101 = Unbundle By Name(w286) -> ("Test Limits"=w288:string[][], "Connect"=w292:string)
        n102 = To Variant(anything=w292) -> (Variant=w289:variant)
        n103 = call "Process Results.vi"("error in (no error)"=w290, "Measurement"=w289, "Test Limits"=w288, "Sub Test Name"=w287) -> ("error out"=w291:errorcluster, "Results Data"=w282:string[])  [unwired: 6 in]
        "Results Data 5" <- w282
        n104 = Build Array (concatenate)(w284, w282) -> (w283:string[][])
        n105 = Bundle By Name(cluster=w286, "Results Data Array"=w283) -> (w285:T5)
        n106 = call <vilib>:"Add State(s) to Queue__jki_lib_state_machine.vi"("State(s) in (\"\")"=w294) -> ("States Out"=w293:string)  [unwired: 14 in]
      }
      frame "---------- Results Data ----------" {
        # "Template Separator\n(You can make a copy of, or modify, this frame)"
        n107 = call <vilib>:"Add State(s) to Queue__jki_lib_state_machine.vi"("State(s) in (\"\")"=w298) -> ("States Out"=w297:string)  [unwired: 14 in]
      }
      frame "Results Data: Write Results Data" {
        w300 = ","  # delimiter (\t)
        w301 = TRUE  # append to file? (new file:F)
        n108 = Unbundle By Name(w303) -> ("Results File Path"=w302:path, "Results Data Array"=w299:string[][])
        "Results Data Array" <- w299
        n109 = call-poly <vilib>:"Write Delimited Spreadsheet.vi"("file path (dialog if empty)"=w302, "2D data"=w299, "append to file? (new file:F)"=w301, "error in (no error)"=w304, "delimiter (\\t)"=w300) -> ("error out"=w305:errorcluster)  [unwired: 9 in, 1 out]
        n110 = call <vilib>:"Add State(s) to Queue__jki_lib_state_machine.vi"("State(s) in (\"\")"=w307) -> ("States Out"=w306:string)  [unwired: 14 in]
      }
      frame "---------- Connect ----------" {
        # "Template Separator\n(You can make a copy of, or modify, this frame)"
        n111 = call <vilib>:"Add State(s) to Queue__jki_lib_state_machine.vi"("State(s) in (\"\")"=w311) -> ("States Out"=w310:string)  [unwired: 14 in]
      }
      frame "Connect: Switch Contactor" {
        # "Template Separator\n(You can make a copy of, or modify, this frame)"
        # "User must set IP address to match this given one"
        n112 = call-poly <vilib>:"DAQmx Create Virtual Channel.vi"("lines"=tag "6525/port0/line0", "error in"=w319) -> ("task out"=w322:refnum<k21>, "error out"=w321:errorcluster)  [unwired: 12 in]
        n113 = call <vilib>:"DAQmx Start Task.vi"("task/channels in"=w322, "error in"=w321) -> ("task out"=w317:refnum<k21>, "error out"=w318:errorcluster)  [unwired: 12 in]
        n114 = call-poly <vilib>:"DAQmx Write.vi"("task/channels in"=w317, "data"=bool[] [TRUE], "error in"=w318) -> ("task out"=w312:refnum<k21>, "error out"=w316:errorcluster)  [unwired: 10 in, 1 out]
        n115 = call <vilib>:"DAQmx Stop Task.vi"("task/channels in"=w312, "error in"=w316) -> ("task out"=w313:refnum<k21>, "error out"=w315:errorcluster)  [unwired: 12 in]
        n116 = call <vilib>:"DAQmx Clear Task.vi"("task in"=w313, "error in"=w315) -> ("error out"=w314:errorcluster)  [unwired: 13 in]
        n117 = call <vilib>:"Add State(s) to Queue__jki_lib_state_machine.vi"("State(s) in (\"\")"=w326) -> ("States Out"=w325:string)  [unwired: 14 in]
      }
      frame "Connect: Set IP Address" {
        # "Template Separator\n(You can make a copy of, or modify, this frame)"
        # "User must set IP address to match this given one"
        n118 = One Button Dialog(message="Make your IP Address 192.168.201.22", button name ("OK")="Done") -> ()  [unwired: 1 out]
        n119 = call <vilib>:"Add State(s) to Queue__jki_lib_state_machine.vi"("State(s) in (\"\")"=w332) -> ("States Out"=w331:string)  [unwired: 14 in]
      }
      frame "Connect: UDP Open" {
        # "If this changes \nchange on CONNECT command as well!"
        # "User must enter their PC IP address"
        # "Open UDP read to RIB box"
        # "Template Separator\n(You can make a copy of, or modify, this frame)"
        # "Open UDP linking to RIB Box."
        n120 = String To IP(1:"192.168.201.22" ("name")) -> (0:w341:u32)
        n121 = UDP Open(7:w341, 8:w340, 11:u16 54321 ("port")) -> (port=w334:refnum<k16>, 0:w336:errorcluster)  [unwired: 2 in, 1 out]
        n122 = call "FGV - Initialise.vi"("Enum"=FGV_-_Enum."Open UDP", "connection ID"=w334, "Error In"=w336) -> ("Error Out"=w335:errorcluster)  [unwired: 9 in, 3 out]
        n123 = Bundle By Name(cluster=w339, "connection ID"=w334) -> (w338:T5)
        n124 = call <vilib>:"Add State(s) to Queue__jki_lib_state_machine.vi"("State(s) in (\"\")"=w344) -> ("States Out"=w343:string)  [unwired: 14 in]
      }
      frame "Connect: I2C Open" {
        # "Template Separator\n(You can make a copy of, or modify, this frame)"
        n125 = call "FGV - Initialise.vi"("Enum"=FGV_-_Enum."Get Data", "Error In"=w346) -> ("task out"=w345:refnum<k21>, "Error Out"=w347:errorcluster)  [unwired: 10 in, 2 out]
        n126 = Bundle By Name(cluster=w350, "task out"=w345) -> (w349:T5)
        n127 = call <vilib>:"Add State(s) to Queue__jki_lib_state_machine.vi"("State(s) in (\"\")"=w352) -> ("States Out"=w351:string)  [unwired: 14 in]
      }
      frame "Connect: UPD Connect Fail" {
        # "Send CONNECT command to RIB Box"
        # "IP for RIB Box is set"
        # "Data"
        # "Length"
        # "ID"
        # "Target"
        # "Type"
        # "Pkt ID"
        # "CONNECT"
        # "Template Separator\n(You can make a copy of, or modify, this frame)"
        n128 = Unbundle By Name(w357) -> ("connection ID"=w356:refnum<k16>)
        n129 = Build Array(u8 91 ("element"), u8 1 ("element"), u8 9 ("element"), u8 1 ("element"), u8 5 ("element"), u8 192 ("element"), u8 168 ("element"), u8 201 ("element"), u8 255 ("element")) -> (w372:u8[])
        n130 = Byte Array To String(unsigned byte array=w372) -> (string=w373:string)
        n131 = String To IP(1:"192.168.201.21" ("name")) -> (0:w361:u32)
        n132 = UDP Write(address=w361, port or service name=u16 54321, connection ID=w356, data in=w373, 8:w358, 9:1000 ("timeout ms (25000)")) -> (error out=w354:errorcluster, 3:w355:refnum<k16>)
        n133 = Bundle By Name(cluster=w357, "connection ID"=w355) -> (w359:T5)
        n134 = Wait (ms)(milliseconds to wait=u32 10) -> ()  [unwired: 1 out]
        n135 = call <vilib>:"Add State(s) to Queue__jki_lib_state_machine.vi"("State(s) in (\"\")"=w376) -> ("States Out"=w375:string)  [unwired: 14 in]
      }
      frame "Connect: Start Timer (Connect Fail)" {
        # "Start 10 second timer"
        # "Template Separator\n(You can make a copy of, or modify, this frame)"
        n136 = call "Timer.vi"("error in (no error)"=w382, "Enum"=T4."Start Timer") -> ("error out"=w378:errorcluster)  [unwired: 6 in, 3 out]
        n137 = property on="Timeout (Connect Fail)" class="Slide (strict)"(error in=w378, "Value"=0.0 ("Horizontal Pointer Slide"), "Maximum"=10.0 ("Target Time"), "Minimum"=0.0 ("Scale.Range:Minimum")) -> (error out=w377:errorcluster)  [unwired: 1 in, 1 out]
        n138 = call <vilib>:"Add State(s) to Queue__jki_lib_state_machine.vi"("State(s) in (\"\")"=w386) -> ("States Out"=w385:string)  [unwired: 14 in]
      }
      frame "Connect: Read Connect Fail" {
        # "Read UDP if equal to F0 test complete if not check if timer has elapsed."
        # "#56 = didnt read before the timeout"
        # "Template Separator\n(You can make a copy of, or modify, this frame)"
        n139 = Unbundle By Name(w412) -> ("connection ID"=w413:refnum<k16>)
        n140 = UDP Read(connection ID=w413, timeout ms (25000)=10, 8:w414) -> (data out=w404:string, error out=w408:errorcluster, 3:w405:refnum<k16>)  [unwired: 1 in, 2 out]
        n141 = String To Byte Array(string=w404) -> (unsigned byte array=w410:u8[])
        n142 = Number To Hexadecimal String(2:w410) -> (0:w397:string[])  [unwired: 1 in]
        n143 = Index Array(array=w397, index #1=0 ("index")) -> (element #1=w398:string, element #2=w402:string, element #3=w401:string, element #4=w400:string, element #5=w399:string, element #6=w396:string, element #7=w395:string, element #8=w394:string, element #9=w393:string)  [unwired: 8 in]
        n144 = Concatenate Strings(w398, w402, w401, w400, w399, w396, w395, w394, w393) -> (w389:string)
        n145 = call <vilib>:"Clear Errors.vi"("error in (no error)"=w408, "specific error code to clear (0: all)"=56) -> ("error out"=w407:errorcluster)  [unwired: 4 in, 1 out]
        n146 = Bundle By Name(cluster=w412, "connection ID"=w405, "Connect Fail"=w389) -> (w411:T5)
        n147 = Equal?(x=w389, y="5B0910") -> (x = y?=w387:bool)
        "Connect Fail" <- w387
        n148 = call-poly <vilib>:"Select State(s)__jki_lib_state_machine.vi"("State(s) if True (\"\")"="Macro: Test 2" ("State(s) if True (\"\")"), "Select"=w387, "State(s) if False (\"\")"="Connect: Elapsed Timer (Connect Fail)" ("State(s) if False (\"\")")) -> ("States Out"=w388:string)  [unwired: 12 in]
        n149 = call <vilib>:"Add State(s) to Queue__jki_lib_state_machine.vi"("State(s) in Front (\"\")"=w388, "State(s) in (\"\")"=w416) -> ("States Out"=w415:string)  [unwired: 13 in]
      }
      frame "Connect: Elapsed Timer (Connect Fail)" {
        # "check if timer elased - if TRUE end test if FALSE read again."
        # "Template Separator\n(You can make a copy of, or modify, this frame)"
        # "Check to see if the timer has elpased."
        n150 = call "Timer.vi"("error in (no error)"=w424, "Target Time"=10.0, "Enum"=T4."Get Time") -> ("error out"=w423:errorcluster, "Time Elapsed?"=w420:bool, "Elapsed Time"=→"Timeout (Connect Fail)":dbl)  [unwired: 5 in, 1 out]
        n151 = call-poly <vilib>:"Select State(s)__jki_lib_state_machine.vi"("State(s) if True (\"\")"="Macro: Test 2" ("State(s) if True (\"\")"), "Select"=w420, "State(s) if False (\"\")"="Connect: Read Connect Fail" ("State(s) if False (\"\")")) -> ("States Out"=w419:string)  [unwired: 12 in]
        n152 = call <vilib>:"Add State(s) to Queue__jki_lib_state_machine.vi"("State(s) in Front (\"\")"=w419, "State(s) in (\"\")"=w428) -> ("States Out"=w427:string)  [unwired: 13 in]
      }
      frame "Connect: UPD Connect" {
        # "Length Wrong to froce a fail!"
        # "Send CONNECT command to RIB Box"
        # "IP for RIB Box is set"
        # "Data"
        # "Length"
        # "ID"
        # "Target"
        # "Type"
        # "Pkt ID"
        # "CONNECT"
        # "Template Separator\n(You can make a copy of, or modify, this frame)"
        n153 = Unbundle By Name(w433) -> ("connection ID"=w432:refnum<k16>)
        n154 = Build Array(u8 91 ("element"), u8 1 ("element"), u8 9 ("element"), u8 1 ("element"), u8 4 ("element"), u8 192 ("element"), u8 168 ("element"), u8 201 ("element"), u8 22 ("element")) -> (w448:u8[])
        n155 = Byte Array To String(unsigned byte array=w448) -> (string=w449:string)
        n156 = String To IP(1:"192.168.201.21" ("name")) -> (0:w437:u32)
        n157 = UDP Write(address=w437, port or service name=u16 54321, connection ID=w432, data in=w449, 8:w434, 9:1000 ("timeout ms (25000)")) -> (error out=w430:errorcluster, 3:w431:refnum<k16>)
        n158 = Bundle By Name(cluster=w433, "connection ID"=w431) -> (w435:T5)
        n159 = Wait (ms)(milliseconds to wait=u32 10) -> ()  [unwired: 1 out]
        n160 = call <vilib>:"Add State(s) to Queue__jki_lib_state_machine.vi"("State(s) in (\"\")"=w452) -> ("States Out"=w451:string)  [unwired: 14 in]
      }
      frame "Connect: Start Timer (Connect)" {
        # "Start 10 second timer"
        # "Template Separator\n(You can make a copy of, or modify, this frame)"
        n161 = call "Timer.vi"("error in (no error)"=w458, "Enum"=T4."Start Timer") -> ("error out"=w454:errorcluster)  [unwired: 6 in, 3 out]
        n162 = property on="Timeout (Connect)" class="Slide (strict)"(error in=w454, "Value"=0.0 ("Horizontal Pointer Slide"), "Maximum"=10.0 ("Target Time"), "Minimum"=0.0 ("Scale.Range:Minimum")) -> (error out=w453:errorcluster)  [unwired: 1 in, 1 out]
        n163 = call <vilib>:"Add State(s) to Queue__jki_lib_state_machine.vi"("State(s) in (\"\")"=w462) -> ("States Out"=w461:string)  [unwired: 14 in]
      }
      frame "Connect: Read Connect" {
        # "Read UDP if equal to F0 test complete if not check if timer has elapsed."
        # "#56 = didnt read before the timeout"
        # "Template Separator\n(You can make a copy of, or modify, this frame)"
        n164 = Unbundle By Name(w488) -> ("connection ID"=w489:refnum<k16>)
        n165 = UDP Read(connection ID=w489, timeout ms (25000)=10, 8:w490) -> (data out=w480:string, error out=w485:errorcluster, 3:w482:refnum<k16>)  [unwired: 1 in, 2 out]
        n166 = String To Byte Array(string=w480) -> (unsigned byte array=w481:u8[])
        n167 = Number To Hexadecimal String(2:w481) -> (0:w469:string[])  [unwired: 1 in]
        n168 = Index Array(array=w469, index #1=0 ("index")) -> (element #1=w474:string, element #2=w478:string, element #3=w477:string, element #4=w476:string, element #5=w475:string, element #6=w473:string, element #7=w472:string, element #8=w471:string, element #9=w470:string)  [unwired: 8 in]
        n169 = Concatenate Strings(w474, w478, w477, w476, w475, w473, w472, w471, w470) -> (w465:string)
        n170 = call <vilib>:"Clear Errors.vi"("error in (no error)"=w485, "specific error code to clear (0: all)"=56) -> ("error out"=w484:errorcluster)  [unwired: 4 in, 1 out]
        n171 = Bundle By Name(cluster=w488, "connection ID"=w482, "Connect"=w465) -> (w487:T5)
        n172 = Equal?(x=w465, y="5B3910") -> (x = y?=w463:bool)
        "Connect" <- w463
        n173 = call-poly <vilib>:"Select State(s)__jki_lib_state_machine.vi"("State(s) if True (\"\")"="Macro: Limits" ("State(s) if True (\"\")"), "Select"=w463, "State(s) if False (\"\")"="Connect: Elapsed Timer (Connect)" ("State(s) if False (\"\")")) -> ("States Out"=w466:string)  [unwired: 12 in]
        n174 = call <vilib>:"Add State(s) to Queue__jki_lib_state_machine.vi"("State(s) in Front (\"\")"=w466, "State(s) in (\"\")"=w492) -> ("States Out"=w491:string)  [unwired: 13 in]
      }
      frame "Connect: Elapsed Timer (Connect)" {
        # "check if timer elased - if TRUE end test if FALSE read again."
        # "Template Separator\n(You can make a copy of, or modify, this frame)"
        # "Check to see if the timer has elpased."
        n175 = call "Timer.vi"("error in (no error)"=w500, "Target Time"=10.0, "Enum"=T4."Get Time") -> ("error out"=w499:errorcluster, "Time Elapsed?"=w496:bool, "Elapsed Time"=→"Timeout (Connect)":dbl)  [unwired: 5 in, 1 out]
        n176 = call-poly <vilib>:"Select State(s)__jki_lib_state_machine.vi"("State(s) if True (\"\")"="Macro: Limits" ("State(s) if True (\"\")"), "Select"=w496, "State(s) if False (\"\")"="Connect: Read Connect" ("State(s) if False (\"\")")) -> ("States Out"=w495:string)  [unwired: 12 in]
        n177 = call <vilib>:"Add State(s) to Queue__jki_lib_state_machine.vi"("State(s) in Front (\"\")"=w495, "State(s) in (\"\")"=w504) -> ("States Out"=w503:string)  [unwired: 13 in]
      }
    }
    n178 = Wait (ms)(milliseconds to wait=u32 2) -> ()  [unwired: 1 out]
  }
  "error out" <- w1
